vi "Check Message Queue Status_sushu.vi"(0 "Queue In":cluster{"Q":T3, "Name":string}, 7 "return elements? (F)":bool, 11 "error in":errorcluster) -> (2 "max queue size":i32, 3 "message queue name":string, 4 "Queue Out":cluster{"Q":T3, "Name":string}, 6 "# elements in queue":i32, 14 "elements":T1[](array[typedef]), 15 "error out":errorcluster)   [LabVIEW 2021]
doc: "Returns the max queue size, message queue name, and the number of elements in the queue."
uses:
  <vilib>/NI/AMC/Message.ctl
  <vilib>/NI/AMC/AMC.lvlib
  <vilib>/NI/AMC/Message Queue.ctl
  <vilib>/NI/Tools/Keyed Array/KeyedArray.ctl
  <vilib>/NI/Tools/Keyed Array/Tools_KeyedArray.lvlib
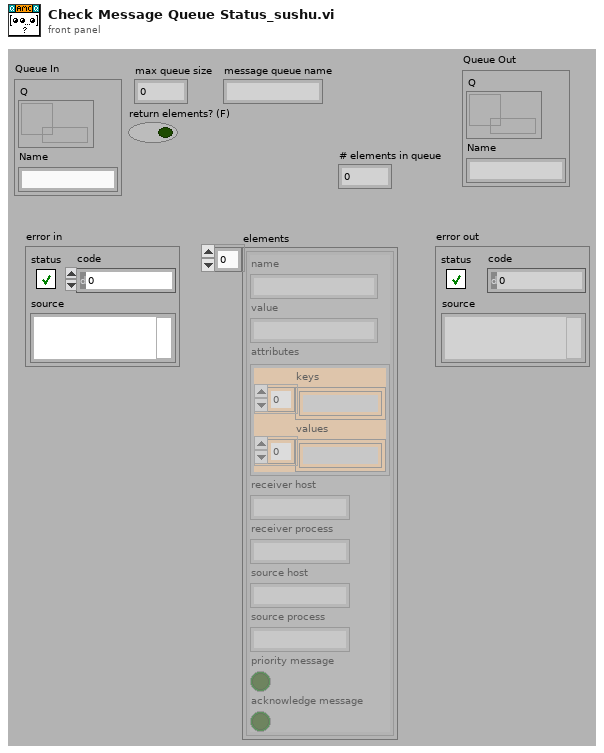
[diagram p1: front panel]
types:
  T1 = typedef "AMC.lvlib/Message.ctl" = cluster{"name":string, "value":string, "attributes":T2, "receiver host":string, "receiver process":string, "source host":string, "source process":string, "priority message":bool, "acknowledge message":bool}
  T2 = typedef "Tools_KeyedArray.lvlib/KeyedArray.ctl" = cluster{"keys":string[], "values":string[]}
  T3 = typedef "AMC.lvlib/Message Queue.ctl" = refnum<queue>
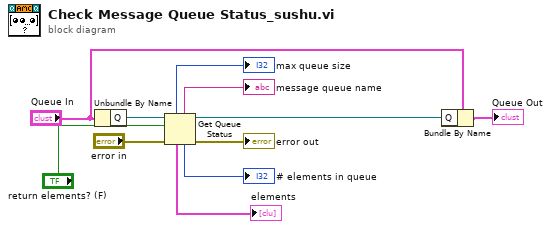
[diagram p0: block diagram]
diagram:
  n1 = Unbundle By Name("Queue In") -> ("Q"=w6:T3)
  n2 = Get Queue Status(queue=w6, return elements? (F)="return elements? (F)", error in (no error)="error in") -> (queue out=w5:T3, queue name=→"message queue name":string, max queue size=→"max queue size":i32, error out=→"error out":errorcluster, # elements in queue=→"# elements in queue":i32, elements=→"elements":T1[])  [unwired: 2 out]
  n3 = Bundle By Name(cluster="Queue In", "Q"=w5) -> (→"Queue Out":cluster{"Q":T3, "Name":string})
